vi "Build TCP String.vi"(11 "Data":string) -> (3 "TCP String":string)   [LabVIEW 2020, in "TCP Send.lvclass"]
uses:
  TCP Send.lvclass
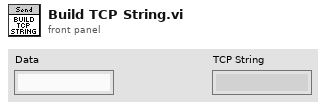
[diagram p1: front panel]
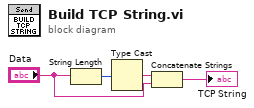
[diagram p0: block diagram]
diagram:
  n1 = String Length(string="Data") -> (length=w3:i32)
  n2 = Type Cast(x=w3) -> (*(type *) &x=w4:string)  [unwired: 1 in]
  n3 = Concatenate Strings(w4, "Data") -> (→"TCP String":string)
